vi "GetChannelValue.vi"(8 "error in (no error)":errorcluster, 10 "#Channel (-1 fo all)":i32, 11 "OXY_SCPI Reseource In":refnum<visa-resource-name>) -> (0 "error out":errorcluster, 1 "communication_data":T1, 2 "Value List":string, 3 "OXY_SCPI Reseource Out":refnum<visa-resource-name>)   [LabVIEW 2018, in "OXYGEN.lvlib"]
doc: "Query Numeric Values of the preset item lists."
uses:
  OXYGEN.lvlib
  TypeDefs/Cluster_RawCommData.ctl
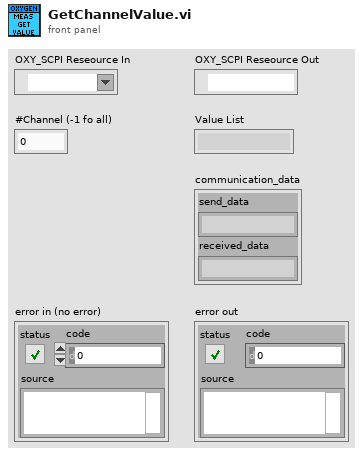
[diagram p1: front panel]
types:
  T1 = typedef "OXYGEN.lvlib/Cluster_RawCommData.ctl" = cluster{"send_data":string, "received_data":string}
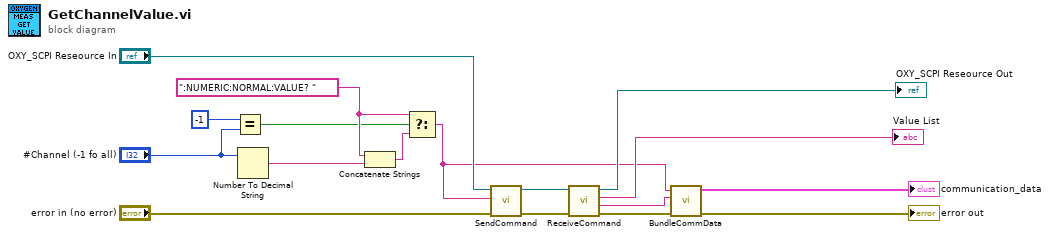
[diagram p0: block diagram]
diagram:
  w6 = ":NUMERIC:NORMAL:VALUE? " ("String to Send")
  n1 = Equal?(x=-1, y="#Channel (-1 fo all)") -> (x = y?=w3:bool)
  n2 = Number To Decimal String(number="#Channel (-1 fo all)") -> (decimal integer string=w11:string)  [unwired: 1 in]
  n3 = Concatenate Strings(w6, w11) -> (w1:string)
  n4 = Select(t=w6, s=w3, f=w1) -> (s? t:f=w5:string)
  n5 = call "SendCommand.vi"("error in (no error)"="error in (no error)", "String to Send"=w5, "OXY_SCPI Reseource In"="OXY_SCPI Reseource In") -> ("error out"=w17:errorcluster, "OXY_SCPI Reseource Out"=w16:refnum<visa-resource-name>)  [unwired: 7 in]
  n6 = call "ReceiveCommand.vi"("error in (no error)"=w17, "OXY_SCPI Reseource In"=w16) -> ("error out"=w14:errorcluster, "received Data with Header"=w7:string, "received Data"=→"Value List":string, "OXY_SCPI Reseource Out"=→"OXY_SCPI Reseource Out":refnum<visa-resource-name>)  [unwired: 6 in]
  n7 = call "BundleCommData.vi"("error in (no error)"=w14, "received_data"=w7, "send_data"=w5) -> ("error out"=→"error out":errorcluster, "communication_data"=→"communication_data":T1)  [unwired: 7 in]
